vi "init.vi"(8 "error in":errorcluster, 10 "UI Reference configuration in":refnum<class "TBM module configuration.lvclass">, 11 "UI Reference runtime in":refnum<class "UI Reference runtime.lvclass">) -> (0 "error out":errorcluster, 1 "data allocations":T1, 2 "execution settings":T4, 3 "UI Reference runtime out":refnum<class "UI Reference runtime.lvclass">)   [LabVIEW 2013, in "UI Reference runtime.lvclass"]
doc: "Provides an interface for initializing a module at runtime. While this interface performs no operations, a child should provide an override which may open any necessary references or sessions, allocate necessary memory, and perform any final configuration validataion before providing the full configuration <b>execution data</b> to the calling process."
uses:
  UI Reference runtime.lvclass
  <vilib>/NI/Tag Bus Module Framework/module configuration/TBM module configuration.lvclass
  <vilib>/NI/Tag Bus Module Framework/runtime/execution settings.ctl
  <vilib>/NI/Tag Bus Module Framework/channel/data tables.ctl
  <vilib>/NI/Tag Bus/dictionary/data dictionary.lvclass
  <vilib>/NI/Tag Bus/dictionary table pair.ctl
  <vilib>/NI/Tag Bus/table/data table.ctl
  configuration/UI Reference configuration.lvclass
  configuration/UI Reference configuration.lvclass/UI Reference configuration.ctl
  UI Reference runtime.lvclass/UI Reference runtime.ctl
  configuration/Read VI Refnum.vi
  configuration/Read VI name.vi
  <vilib>/NI/Tag Bus Module Framework/channel/TBM channel.lvclass
  <vilib>/NI/Tag Bus Module Framework/runtime/TBM module execution interface.lvclass
  <vilib>/NI/Tag Bus/tag bus.lvlib
  <vilib>/NI/Tag Bus/table/data table.lvlib
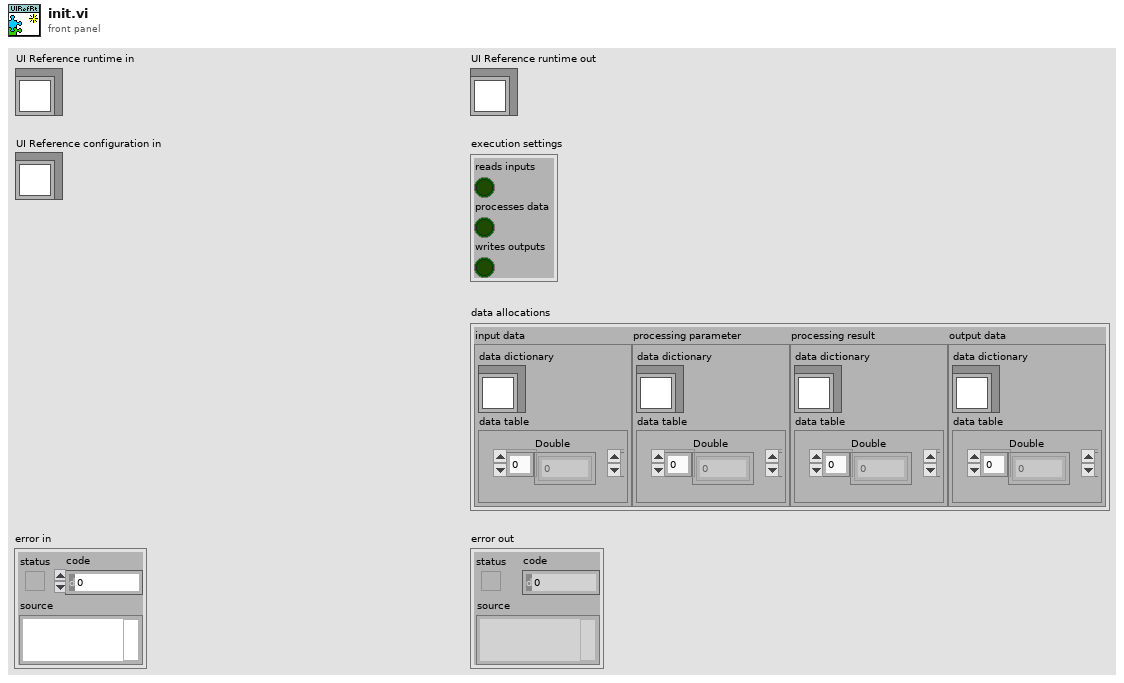
[diagram p1: front panel]
types:
  T1 = typedef "TBM channel.lvclass/data tables.ctl" = cluster{"input data":T2, "processing parameter":T2, "processing result":T2, "output data":T2}
  T2 = typedef "tag bus.lvlib/dictionary table pair.ctl" = cluster{"data dictionary":refnum<class "data dictionary.lvclass">, "data table":T3}
  T3 = typedef "tag bus.lvlib/data table.lvlib/data table.ctl" = cluster{"Double":dbl[], "Single":sgl[], "I64":i64[], "I32":i32[], "I16":i16[], "I8":i8[], "U64":u64[], "U32":u32[], "U16":u16[], "U8":u8[], "Boolean":bool[], "String":string[], "Array of Double":cluster{"DBL Array":dbl[]}[], "Array of Single":cluster{"SGL Array":sgl[]}[], "Array of I64":cluster{"I64 Array":i64[]}[], "Array of I32":cluster{"I32 Array":i32[]}[], "Array of I16":cluster{"I16 Array":i16[]}[], "Array of I8":cluster{"I8 Array":i8[]}[], "Array of U64":cluster{"U64 Array":u64[]}[], "Array of U32":cluster{"U32 Array":u32[]}[], "Array of U16":cluster{"U16 Array":u16[]}[], "Array of U8":cluster{"U8 Array":u8[]}[], "Array of Boolean":cluster{"Boolean Array":bool[]}[], "Array of String":cluster{"String Array":string[]}[]}
  T4 = typedef "TBM module execution interface.lvclass/execution settings.ctl" = cluster{"reads inputs":bool, "processes data":bool, "writes outputs":bool}
  T5 = typedef "UI Reference runtime.lvclass/control index set.ctl" = cluster{"data type":T6, "control indexes":i32[], "data indexes":i32[]}
  T6 = typedef "tag bus.lvlib/tag descriptor.lvclass/Data Type.ctl" = enum16{"Double", "Single", "I64", "I32", "I16", "I8", "U64", "U32", "U16", "U8", "Boolean", "String", "Array of Double", "Array of Single", "Array of I64", "Array of I32", "Array of I16", "Array of I8", "Array of U64", "Array of U32", "Array of U16", "Array of U8", "Array of Boolean", "Array of String"}
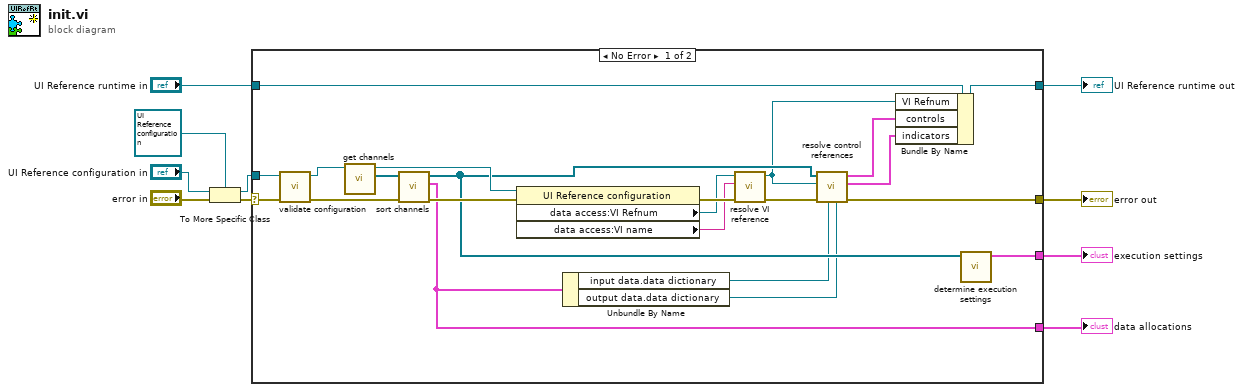
[diagram p0: block diagram]
diagram:
  n1 = To More Specific Class(target class=refnum<class "UI Reference configuration.lvclass"> refnum ("Synchronous module configuration"), reference="UI Reference configuration in", error in="error in") -> (specific class reference=w9:refnum<class "UI Reference configuration.lvclass">, error out=w10:errorcluster)
  n2 = case shown="No Error" w10 {
    selector: w10 -> [w28 w33]
    tunnel: w9 -> [w27 _]
    tunnel: "UI Reference runtime in" -> [w32 w34]
    tunnel: [w20 w34] -> w4
    tunnel: [w19 w33] -> w3
    tunnel: [w13 _] -> w1
    tunnel: [w30 _] -> w2
    frame No Error {
      n3 = call-dynamic "validate configuration.vi"("error in"=w28, "UI Reference configuration in"=w27) -> ("error out"=w29:errorcluster, "UI Reference configuration out"=w26:refnum<class "UI Reference configuration.lvclass">)  [unwired: 8 in]
      n4 = call-dynamic "get channels.vi"("UI Reference configuration in"=w26) -> ("channels"=w25:refnum<class "TBM channel.lvclass">[], "UI Reference configuration out"=w24:refnum<class "UI Reference configuration.lvclass">)  [unwired: 9 in]
      n5 = call <vilib>:"sort channels.vi"("error in"=w29, "channels in"=w25) -> ("error out"=w31:errorcluster, "data allocations"=w13:T1, "channels out"=w15:refnum<class "TBM channel.lvclass">[])  [unwired: 7 in]
      n6 = property class="UI Reference configuration"(reference=w24, error in=w31) -> (error out=w23:errorcluster, "data access:VI Refnum"=w22:refnum<vi>, "data access:VI name"=w21:string)  [unwired: 1 out]
      n7 = Unbundle By Name(w13) -> ("input data.data dictionary"=w11:refnum<class "data dictionary.lvclass">, "output data.data dictionary"=w12:refnum<class "data dictionary.lvclass">)
      n8 = call "resolve VI reference.vi"("error in"=w23, "VI name"=w21, "VI reference"=w22) -> ("error out"=w18:errorcluster, "UI Ref"=w14:refnum<vi>)  [unwired: 7 in]
      n9 = call "resolve control references.vi"("output dictionary"=w12, "input dictionary"=w11, "error in"=w18, "UI Ref"=w14, "channels in"=w15) -> ("error out"=w19:errorcluster, "indicators"=w17:T5[], "controls"=w16:T5[])  [unwired: 4 in]
      n10 = Bundle By Name(cluster=w32, "VI Refnum"=w14, "controls"=w16, "indicators"=w17) -> (w20:refnum<class "UI Reference runtime.lvclass">)
      n11 = call <vilib>:"determine execution settings.vi"("channels"=w15) -> ("execution settings"=w30:T4)  [unwired: 10 in]
    }
    frame Error {
    }
  }
  "error out" <- w3
  "UI Reference runtime out" <- w4
  "execution settings" <- w2
  "data allocations" <- w1
